vi "Modify Run-Time Menu for Spectral Graph.vi"(7 "spectra info":T1[](array[typedef]) {"x-axis units" items=["Time (s)"=0, "Frequency-CB (Hz)"=1, "Frequency-CPB (Hz)"=1248, "Frequency-Arbitrary (Hz)"=2357, "Quefrency (s)"=2, "Revolutions (rev)"=3, "Order"=4, "Speed (RPM)"=11, "Speed (rad/s)"=21, "Index"=65535]; "weighting filter" items=["Linear", "A-weighting", "B-weighting", "C-weighting", "ITU-R 468-4", "Dolby", "CCITT", "C-message", "Wb", "Wc", "Wd", "We", "Wf", "Wh", "Wj", "Wk", "Wm", "AES17 20 kHz lowpass", "AES17 40 kHz lowpass", "AES17 20 kHz highpass", "AES17 40 kHz highpass"]; "dB reference [EU]" format="%.2f"; "engineering units" items=["custom..."=0, "V"=1, "A"=21, "C"=30, "pC"=31, "s"=32, "-"=29, "Pa"=2, "N"=20, "g"=3, "m/s^2"=4, "m/s"=5, "m"=6, "mm/s"=12, "mm"=13, "micron/s"=14, "micron"=15, "in/s^2"=7, "in/s"=8, "in"=9, "mil/s"=10, "mil"=11, "rad/s^2"=16, "rad/s"=17, "rad"=18, "deg/s^2"=26, "deg/s"=27, "deg"=28, "RPM"=22, "cycle/s^2"=23, "Hz"=24, "cycle"=25, "strain"=19]; "spectral info"."window" items=["None "=0, "Hanning"=1, "Hamming"=2, "Blackman-Harris"=3, "Exact Blackman"=4, "Blackman"=5, "Flat Top"=6, "4 Term B-Harris "=7, "7 Term B-Harris"=8, "Low Sidelobe"=9, "Force - Exponential"=10, "Gaussian"=62]}, 10 "Menu in":refnum<k9>, 11 "Display State In":T7={"Graph Visible Items"={"Plot Legend"=FALSE, "Scale Legend"=FALSE, "Graph Palette"=FALSE, "Cursor Legend"=FALSE, "X Scrollbar"=FALSE}, "View Table"=FALSE, "Table Visible Items"={"Vertical Scrollbar"=FALSE, "Horizontal Scrollbar"=FALSE, "Row Headers"=FALSE, "Column Headers"=FALSE, "Vertical Lines"=FALSE, "Horizontal Lines"=FALSE}, "Header Font"={"Font Name"="", "Size"=0, "Bold"=FALSE, "Italic"=FALSE, "Underline"=FALSE, "Strikeout"=FALSE, "Color"=0}, "Cell Font"={"Font Name"="", "Size"=0, "Bold"=FALSE, "Italic"=FALSE, "Underline"=FALSE, "Strikeout"=FALSE, "Color"=0}, "Description and Tip..."={"Description"="", "Tip"=""}, "Moveable Splitter Position"=0, "Measurement Cursor Configuration"={"XY"={"enable XY"=FALSE, "Position (X)"=[], "Type"=enum."Absolute", "Y reference"=0.0, "color"=0}, "band"={"enable band"=FALSE, "B1"=0.0, "B2"=0.0, "Fixed bandwidth (B2-B1)"=0.0, "B1 color"=0, "B2 color"=0}, "harmonic"={"enable harmonics"=FALSE, "X reference (1X)"=0.0, "Maximum"=0, "Subset"=enum."All", "1X color"=0, "MX color"=0}, "sideband"={"enable sideband"=FALSE, "X center (C)"=0.0, "Sidebands"=0, "X spacing (s)"=0.0, "Center color"=0, "Sideband color"=0}}, "Cursors"={"List"=[], "Tags"=[]}, "X Increment"=0.0, "X Scale"={"Label Visible"=FALSE, "Label Text"="", "Mapping Mode"=0, "Format String"=""}, "Y Scale"={"Label Visible"=FALSE, "Label Text"="", "Mapping Mode"=0, "Format String"=""}, "Colors"={"background"=16777215, "major grid"=8355711, "minor grid"=12632256, "font"=0}, "desired spectrum view"={"scaling"={"linear/dB"=enum."no change", "dB reference"=0.0, "power/magnitude"=enum."no change", "view"=enum."no change"}, "spectral density"=enum."no change"}, "Plot Color Wheel"=[3381759, 32768, 982784, 4375295, 13827953, 13457919, 16757522, 4343295, 16728758, 12095254], "Plots"=[], "registered user events"=variant, "Lock 1X to Peak"=FALSE, "spectrum component"=32, "phase spectrum view"={"desired units"=0, "desired wrapping"=4}} caption="State" {"phase spectrum view"."desired wrapping" items=["No change", "Unwrap", "Wrap: -360 to 0", "Wrap: -270 to 90", "Wrap: -180 to 180", "Wrap: -90 to 270", "Wrap: 0 to 360", "Wrap: custom range"]; "phase spectrum view"."desired units" items=["No change", "Radians", "Degrees", "Cycles"]; "spectrum component" items=["Magnitude^2"=37, "Magnitude"=32, "Phase"=33, "Real"=34, "Imaginary"=35, "Coherence"=36, "Unknown"=99]; "Y Scale"."Mapping Mode" items=["Linear", "Logarithmic", "dB"]; "X Scale"."Mapping Mode" items=["Linear", "Logarithmic"]}) -> (3 "Display State out":T7={"Graph Visible Items"={"Plot Legend"=FALSE, "Scale Legend"=FALSE, "Graph Palette"=FALSE, "Cursor Legend"=FALSE, "X Scrollbar"=FALSE}, "View Table"=FALSE, "Table Visible Items"={"Vertical Scrollbar"=FALSE, "Horizontal Scrollbar"=FALSE, "Row Headers"=FALSE, "Column Headers"=FALSE, "Vertical Lines"=FALSE, "Horizontal Lines"=FALSE}, "Header Font"={"Font Name"="", "Size"=0, "Bold"=FALSE, "Italic"=FALSE, "Underline"=FALSE, "Strikeout"=FALSE, "Color"=0}, "Cell Font"={"Font Name"="", "Size"=0, "Bold"=FALSE, "Italic"=FALSE, "Underline"=FALSE, "Strikeout"=FALSE, "Color"=0}, "Description and Tip..."={"Description"="", "Tip"=""}, "Moveable Splitter Position"=0, "Measurement Cursor Configuration"={"XY"={"enable XY"=FALSE, "Position (X)"=[], "Type"=enum."Absolute", "Y reference"=0.0, "color"=0}, "band"={"enable band"=FALSE, "B1"=0.0, "B2"=0.0, "Fixed bandwidth (B2-B1)"=0.0, "B1 color"=0, "B2 color"=0}, "harmonic"={"enable harmonics"=FALSE, "X reference (1X)"=0.0, "Maximum"=0, "Subset"=enum."All", "1X color"=0, "MX color"=0}, "sideband"={"enable sideband"=FALSE, "X center (C)"=0.0, "Sidebands"=0, "X spacing (s)"=0.0, "Center color"=0, "Sideband color"=0}}, "Cursors"={"List"=[], "Tags"=[]}, "X Increment"=0.0, "X Scale"={"Label Visible"=FALSE, "Label Text"="", "Mapping Mode"=0, "Format String"=""}, "Y Scale"={"Label Visible"=FALSE, "Label Text"="", "Mapping Mode"=0, "Format String"=""}, "Colors"={"background"=16777215, "major grid"=8355711, "minor grid"=12632256, "font"=0}, "desired spectrum view"={"scaling"={"linear/dB"=enum."no change", "dB reference"=0.0, "power/magnitude"=enum."no change", "view"=enum."no change"}, "spectral density"=enum."no change"}, "Plot Color Wheel"=[3381759, 32768, 982784, 4375295, 13827953, 13457919, 16757522, 4343295, 16728758, 12095254], "Plots"=[], "registered user events"=variant, "Lock 1X to Peak"=FALSE, "spectrum component"=32, "phase spectrum view"={"desired units"=0, "desired wrapping"=4}} caption="State" {"phase spectrum view"."desired wrapping" items=["No change", "Unwrap", "Wrap: -360 to 0", "Wrap: -270 to 90", "Wrap: -180 to 180", "Wrap: -90 to 270", "Wrap: 0 to 360", "Wrap: custom range"]; "phase spectrum view"."desired units" items=["No change", "Radians", "Degrees", "Cycles"]; "spectrum component" items=["Magnitude^2"=37, "Magnitude"=32, "Phase"=33, "Real"=34, "Imaginary"=35, "Coherence"=36, "Unknown"=99]; "Y Scale"."Mapping Mode" items=["Linear", "Logarithmic", "dB"]; "X Scale"."Mapping Mode" items=["Linear", "Logarithmic"]})   [LabVIEW 2017, in "Spectrum with Cursors.xctl"]
uses:
  <vilib>/addons/_XControls/Spectrum with Cursors/Spectrum with Cursors.xctl
  <vilib>/addons/_XControls/Spectrum with Cursors/Controls/State.ctl
  <vilib>/Utility/miscctls.llb/LVFontTypeDef.ctl
  <vilib>/addons/_XControls/Spectrum with Cursors/Controls/Measurement Cursor Configuration.ctl
  <vilib>/addons/_NISVFA/_Shared subVIs/Controls/NI Spectrum Component.ctl
  <vilib>/addons/_NISVFA/_Shared subVIs/Controls/svc_Spectrum Info.ctl
  <vilib>/addons/_NISVFA/_Shared subVIs/Controls/svc_X-Axis Units.ctl
  <vilib>/addons/_NISVFA/_Shared subVIs/Controls/svc_Spectrum Type.ctl
  <vilib>/addons/_NISVFA/_Shared subVIs/Controls/svc_Engineering Units Text Ring.ctl
  <vilib>/addons/_NISVFA/_Shared subVIs/Controls/svc_Weighting Filter Text Ring.ctl
  <vilib>/addons/_NISVFA/_Shared subVIs/Controls/svc_Complimentary Spectrum Units.ctl
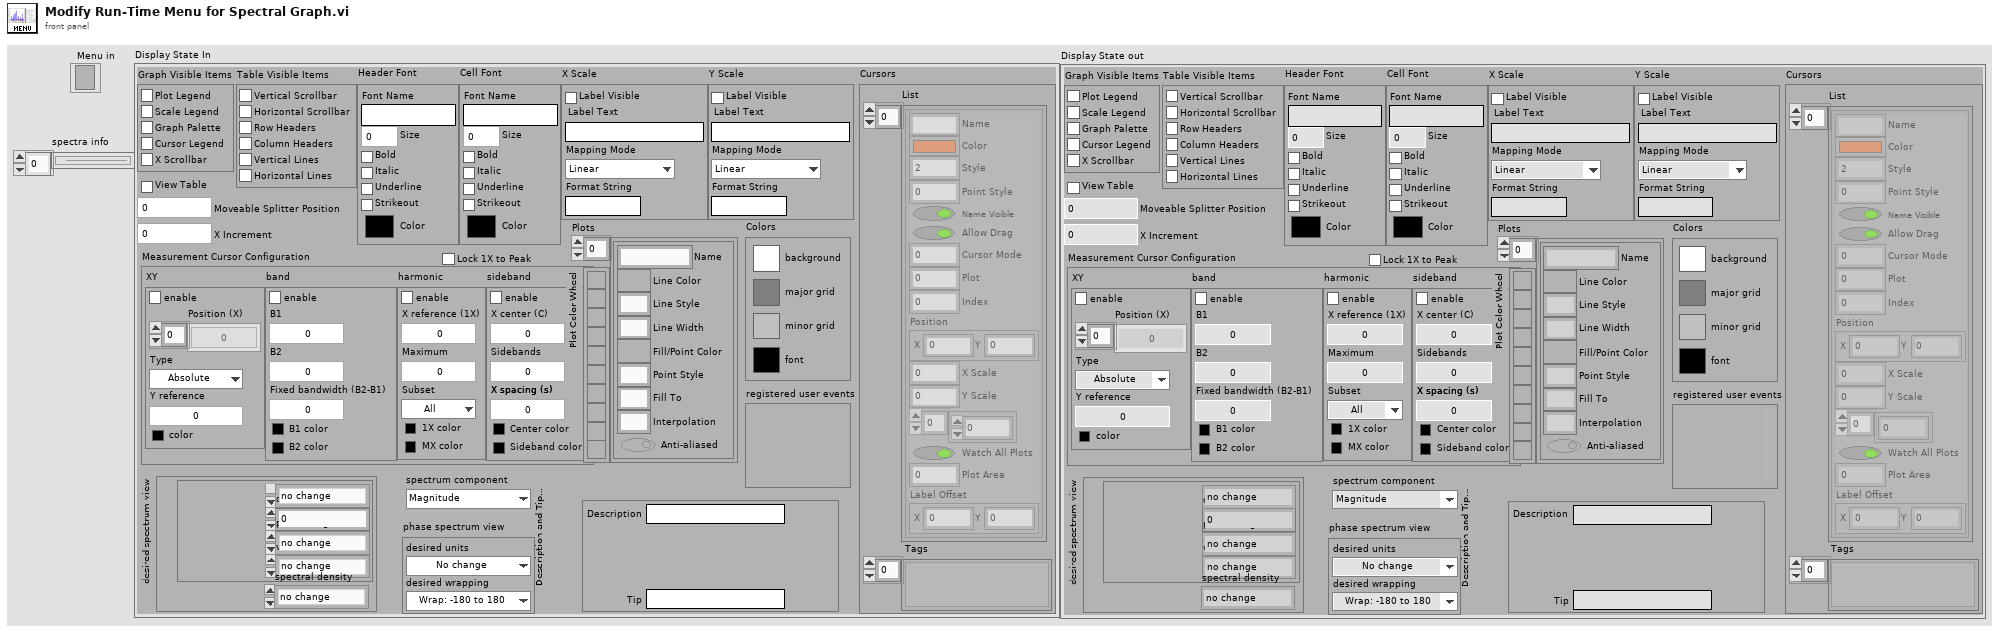
[diagram p1: front panel]
types:
  T1 = typedef "svc_Spectrum Info.ctl" = cluster{"channel name":string, "description":string, "x-axis units":T2, "spectral info":cluster{"spectrum type":T3, "linear/dB":enum16{"linear", "dB"}, "window":u16, "window size":i32, "FFT size":i32}, "engineering units":T4, "custom label":string, "dB reference [EU]":dbl, "peak units":enum16{"rms", "peak", "peak-peak"}, "weighting filter":T5, "spectral density?":bool, "unit label":string, "spectrum skewed?":bool, "complimentary spectrum units":T6}
  T2 = typedef "svc_X-Axis Units.ctl" = u16
  T3 = typedef "svc_Spectrum Type.ctl" = enum16{"FFT Spectrum [complex]", "Amplitude [Magnitude]", "Power [Magnitude^2]", "Cross Spectrum [complex]", "Frequency Response [Complex]"}
  T4 = typedef "svc_Engineering Units Text Ring.ctl" = u16
  T5 = typedef "svc_Weighting Filter Text Ring.ctl" = u16
  T6 = typedef "svc_Complimentary Spectrum Units.ctl" = enum16{"none", "radians", "degrees", "cycles", "imaginary"}
  T7 = typedef "Spectrum with Cursors.xctl/State.ctl" = cluster{"Graph Visible Items":cluster{"Plot Legend":bool, "Scale Legend":bool, "Graph Palette":bool, "Cursor Legend":bool, "X Scrollbar":bool}, "View Table":bool, "Table Visible Items":cluster{"Vertical Scrollbar":bool, "Horizontal Scrollbar":bool, "Row Headers":bool, "Column Headers":bool, "Vertical Lines":bool, "Horizontal Lines":bool}, "Header Font":T8, "Cell Font":T8, "Description and Tip...":cluster{"Description":string, "Tip":string}, "Moveable Splitter Position":i32, "Measurement Cursor Configuration":T9, "Cursors":cluster{"List":cluster{"Name":string, "Color":u32, "Style":i32, "Point Style":u8, "Name Visible":bool, "Allow Drag":bool, "Cursor Mode":u32, "Plot":i32, "Index":i32, "Position":cluster{"X":dbl, "Y":dbl}, "X Scale":u32, "Y Scale":u32, "Watch Plots":i32[], "Watch All Plots":bool, "Plot Area":i32, "Label Offset":cluster{"X":dbl, "Y":dbl}}[], "Tags":variant[]}, "X Increment":dbl, "X Scale":cluster{"Label Visible":bool, "Label Text":string, "Mapping Mode":u8, "Format String":string}, "Y Scale":cluster{"Label Visible":bool, "Label Text":string, "Mapping Mode":u8, "Format String":string}, "Colors":cluster{"background":u32, "major grid":u32, "minor grid":u32, "font":u32}, "desired spectrum view":cluster{"scaling":cluster{"linear/dB":enum16{"no change", "linear", "dB"}, "dB reference":dbl, "power/magnitude":enum16{"no change", "power", "magnitude"}, "view":enum16{"no change", "rms", "peak", "peak-peak"}}, "spectral density":enum16{"no change", "spectrum", "spectral density"}}, "Plot Color Wheel":u32[], "Plots":cluster{"Name":string, "Line Color":u32, "Line Style":u8, "Line Width":u8, "Fill/Point Color":u32, "Point Style":u8, "Fill To":i16, "Interpolation":u8, "Anti-aliased":bool}[], "registered user events":variant, "Lock 1X to Peak":bool, "spectrum component":T10, "phase spectrum view":cluster{"desired units":u16, "desired wrapping":u16}}
  T8 = typedef "LVFontTypeDef.ctl" = cluster{"Font Name":string, "Size":u16, "Bold":bool, "Italic":bool, "Underline":bool, "Strikeout":bool, "Color":u32}
  T9 = typedef "Spectrum with Cursors.xctl/Measurement Cursor Configuration.ctl" = cluster{"XY":cluster{"enable XY":bool, "Position (X)":dbl[], "Type":enum16{"Absolute", "Relative"}, "Y reference":dbl, "color":u32}, "band":cluster{"enable band":bool, "B1":dbl, "B2":dbl, "Fixed bandwidth (B2-B1)":dbl, "B1 color":u32, "B2 color":u32}, "harmonic":cluster{"enable harmonics":bool, "X reference (1X)":dbl, "Maximum":i32, "Subset":enum16{"All", "Even", "Odd"}, "1X color":u32, "MX color":u32}, "sideband":cluster{"enable sideband":bool, "X center (C)":dbl, "Sidebands":i32, "X spacing (s)":dbl, "Center color":u32, "Sideband color":u32}}
  T10 = typedef "NI Spectrum Component.ctl" = u16
  T11 = enum16{"no change", "spectrum", "spectral density"}
  T12 = enum16{"No change", "Radians", "Degrees", "Cycles"}
  T13 = enum16{"No change", "Unwrap", "Wrap: -360 to 0", "Wrap: -270 to 90", "Wrap: -180 to 180", "Wrap: -90 to 270", "Wrap: 0 to 360", "Wrap: custom range"}
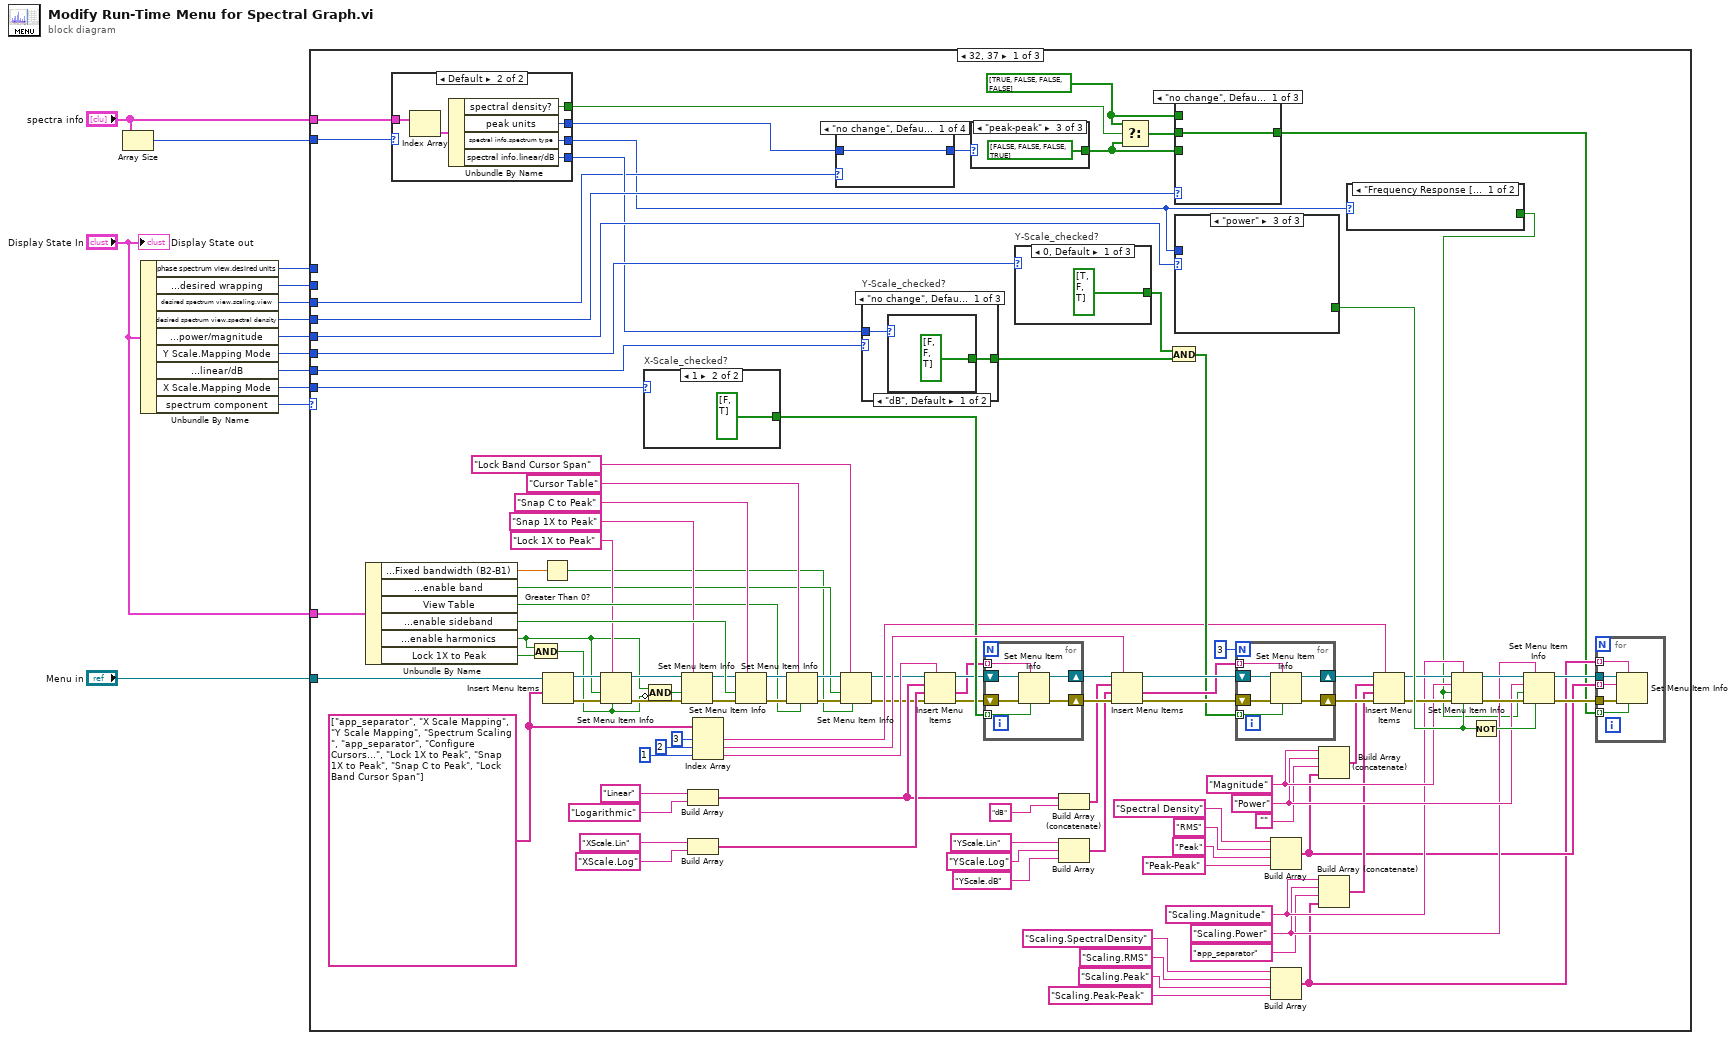
[diagram p0: block diagram]
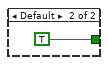
[diagram p2: hidden frame]
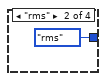
[diagram p3: hidden frame]
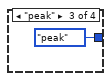
[diagram p4: hidden frame]
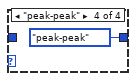
[diagram p5: hidden frame]
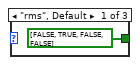
[diagram p6: hidden frame]
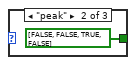
[diagram p7: hidden frame]
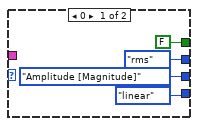
[diagram p8: hidden frame]
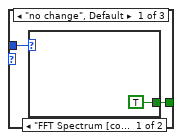
[diagram p11: hidden frame]
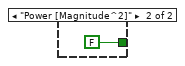
[diagram p12: hidden frame]
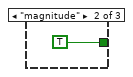
[diagram p13: hidden frame]
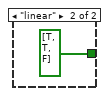
[diagram p14: hidden frame]
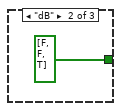
[diagram p15: hidden frame]
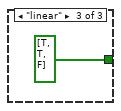
[diagram p16: hidden frame]
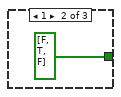
[diagram p17: hidden frame]
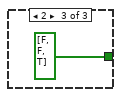
[diagram p18: hidden frame]
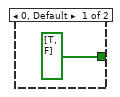
[diagram p19: hidden frame]
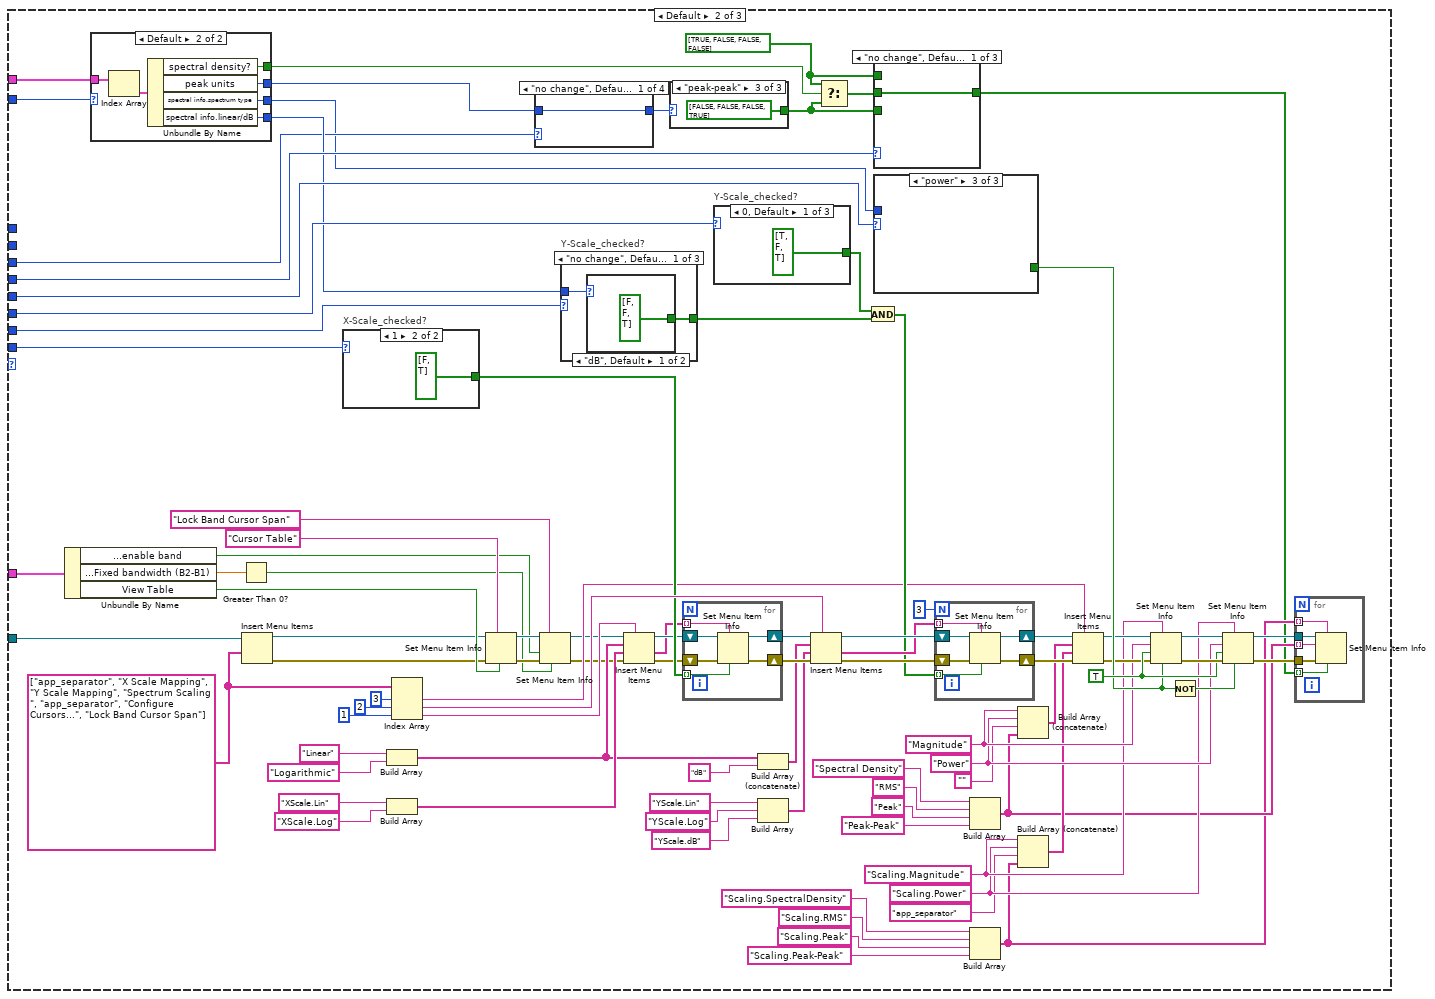
[diagram p20: hidden frame]
diagram:
  n1 = Array Size(array="spectra info") -> (size(s)=w6:i32)
  n2 = Unbundle By Name("Display State In") -> ("phase spectrum view.desired units"=w2:u16, "phase spectrum view.desired wrapping"=w1:u16, "desired spectrum view.scaling.view"=w4:enum16{"no change", "rms", "peak", "peak-peak"}, "desired spectrum view.spectral density"=w7:T11, "desired spectrum view.scaling.power/magnitude"=w8:enum16{"no change", "power", "magnitude"}, "Y Scale.Mapping Mode"=w10:u8, "desired spectrum view.scaling.linear/dB"=w9:enum16{"no change", "linear", "dB"}, "X Scale.Mapping Mode"=w12:u8, "spectrum component"=w3:T10)
  n3 = case shown="32, 37" w3 {
    tunnel: "Menu in" -> [w112 w265 w386]
    tunnel: w12 -> [w103 w256 w377]
    tunnel: "Display State In" -> [w97 w250 w371]
    tunnel: w10 -> [w96 w249 _]
    tunnel: w9 -> [w80 w233 _]
    tunnel: w8 -> [w64 w225 _]
    tunnel: w7 -> [w45 w206 _]
    tunnel: w6 -> [w44 w205 w336]
    tunnel: "spectra info" -> [w43 w204 w337]
    tunnel: w4 -> [w27 w188 _]
    tunnel: w2 -> [_ _ w322]
    tunnel: w1 -> [_ _ w324]
    frame 32, 37 {
      w29 = bool[] [TRUE, FALSE, FALSE, FALSE]
      w51 = "Scaling.Power"
      w52 = "Scaling.Magnitude"
      w54 = "Power" ("element")
      w55 = "Magnitude" ("element")
      w107 = string[] ["app_separator", "X Scale Mapping", "Y Scale Mapping", "Spectrum Scaling ", "app_separator", "Configure Cursors...", "Lock 1X to Peak", "Snap 1X to Peak", "Snap C to Peak", "Lock Band Cursor Span"]
      n4 = Unbundle By Name(w97) -> ("Measurement Cursor Configuration.band.Fixed bandwidth (B2-B1)"=w17:dbl, "Measurement Cursor Configuration.band.enable band"=w18:bool, "View Table"=w110:bool, "Measurement Cursor Configuration.sideband.enable sideband"=w119:bool, "Measurement Cursor Configuration.harmonic.enable harmonics"=w69:bool, "Lock 1X to Peak"=w71:bool)
      n5 = case shown="Default" w44 {
        tunnel: w43 -> [_ w142]
        tunnel: [enum16{"rms", "peak", "peak-peak"}."rms" ("peak units") w140] -> w26
        tunnel: [FALSE ("spectral density?") w137] -> w30
        tunnel: [svc_Spectrum_Type."Amplitude [Magnitude]" ("spectrum type") w139] -> w15
        tunnel: [enum16{"linear", "dB"}."linear" ("linear/dB") w138] -> w42
        frame 0 {
        }
        frame Default {
          n6 = Index Array(array=w142) -> (element=w141:T1)  [unwired: 1 in]
          n7 = Unbundle By Name(w141) -> ("spectral density?"=w137:bool, "peak units"=w140:enum16{"rms", "peak", "peak-peak"}, "spectral info.spectrum type"=w139:T3, "spectral info.linear/dB"=w138:enum16{"linear", "dB"})
        }
      }
      n8 = And(x=w69, y=w71) -> (x .and. y?=w70:bool)
      n9 = Greater Than 0?(x=w17) -> (x > 0?=w16:bool)
      n10 = Insert Menu Items(7:w107, 9:w112) -> (0:w73:errorcluster, 3:w74:refnum<k9>)  [unwired: 4 in, 1 out]
      n11 = Set Menu Item Info(6:w70, 7:"Lock 1X to Peak", 8:w73, 9:w69, 11:w74) -> (0:w76:errorcluster, 3:w75:refnum<k9>)  [unwired: 2 in]
      n12 = case "X-Scale_checked?" shown="1" w103 {
        tunnel: [bool[] [TRUE, FALSE] bool[] [FALSE, TRUE]] -> w95
        frame 0, Default {
        }
        frame 1 {
        }
      }
      n13 = Compound Arithmetic op=AND(w69, invert w70) -> (w68:bool)
      n14 = Set Menu Item Info(7:"Snap 1X to Peak", 8:w76, 9:w68, 11:w75) -> (0:w116:errorcluster, 3:w113:refnum<k9>)  [unwired: 3 in]
      n15 = Build Array("Linear", "Logarithmic") -> (w84:string[])
      n16 = Build Array("XScale.Lin", "XScale.Log") -> (w89:string[])
      n17 = Index Array(array=w107, index #1=3 ("index"), index #2=2 ("index"), index #3=1 ("index")) -> (element #1=w56:string, element #2=w104:string, element #3=w92:string)
      n18 = Set Menu Item Info(7:"Snap C to Peak", 8:w116, 9:w119, 11:w113) -> (0:w115:errorcluster, 3:w114:refnum<k9>)  [unwired: 3 in]
      n19 = Set Menu Item Info(6:w110, 7:"Cursor Table", 8:w115, 11:w114) -> (0:w23:errorcluster, 3:w22:refnum<k9>)  [unwired: 3 in]
      n20 = case shown="\"no change\", Default" w27 {
        tunnel: w26 -> [w121 _ _ _]
        tunnel: [w121 enum16{"rms", "peak", "peak-peak"}."rms" ("peak units") enum16{"rms", "peak", "peak-peak"}."peak" ("peak units") enum16{"rms", "peak", "peak-peak"}."peak-peak" ("peak units")] -> w25
        frame "no change", Default {
        }
        frame "rms" {
        }
        frame "peak" {
        }
        frame "peak-peak" {
        }
      }
      n21 = Set Menu Item Info(6:w16, 7:"Lock Band Cursor Span", 8:w23, 9:w18, 11:w22) -> (0:w20:errorcluster, 3:w21:refnum<k9>)  [unwired: 2 in]
      n22 = case "Y-Scale_checked?" shown="\"no change\", Default" w80 {
        tunnel: [w152 bool[] [FALSE, FALSE, TRUE] bool[] [TRUE, TRUE, FALSE]] -> w79
        tunnel: w42 -> [w151 _ _]
        frame "no change", Default {
          n23 = case shown="\"dB\", Default" w151 {
            tunnel: [bool[] [FALSE, FALSE, TRUE] bool[] [TRUE, TRUE, FALSE]] -> w152
            frame "dB", Default {
            }
            frame "linear" {
            }
          }
        }
        frame "dB" {
        }
        frame "linear" {
        }
      }
      n24 = Insert Menu Items(5:w92, 6:w20, 7:w89, 8:w84, 9:w21) -> (0:w93:errorcluster, 1:w88:string[], 3:w94:refnum<k9>)  [unwired: 1 in]
      n25 = case shown="\"peak-peak\"" w25 {
        tunnel: [bool[] [FALSE, TRUE, FALSE, FALSE] bool[] [FALSE, FALSE, TRUE, FALSE] bool[] [FALSE, FALSE, FALSE, TRUE]] -> w24
        frame "rms", Default {
        }
        frame "peak" {
        }
        frame "peak-peak" {
        }
      }
      n26 = for {
        shift-right: [w166] -> w101
        shift-left: w94 -> [w168]
        shift-right: [w165] -> w102
        shift-left: w93 -> [w167]
        tunnel: w95 -> [w164] mode=indexing
        tunnel: w88 -> [w163] mode=indexing
        n27 = Set Menu Item Info(6:w164, 7:w163, 8:w167, 11:w168) -> (0:w165:errorcluster, 3:w166:refnum<k9>)  [unwired: 3 in]
      }
      n28 = case "Y-Scale_checked?" shown="0, Default" w96 {
        tunnel: [bool[] [TRUE, FALSE, TRUE] bool[] [FALSE, TRUE, FALSE] bool[] [FALSE, FALSE, TRUE]] -> w77
        frame 0, Default {
        }
        frame 1 {
        }
        frame 2 {
        }
      }
      n29 = Build Array (concatenate)(w84, "dB") -> (w83:string[])
      n30 = Build Array("YScale.Lin", "YScale.Log", "YScale.dB") -> (w85:string[])
      n31 = Insert Menu Items(5:w104, 6:w102, 7:w85, 8:w83, 9:w101) -> (0:w99:errorcluster, 1:w98:string[], 3:w100:refnum<k9>)  [unwired: 1 in]
      n32 = Select(t=w29, s=w30, f=w24) -> (s? t:f=w28:bool[])
      n33 = And(x=w77, y=w79) -> (x .and. y?=w78:bool[])
      n34 = case shown="\"no change\", Default" w45 {
        tunnel: [w143 w144 w145] -> w31
        tunnel: w29 -> [_ _ w145]
        tunnel: w28 -> [w143 _ _]
        tunnel: w24 -> [_ w144 _]
        frame "no change", Default {
        }
        frame "spectrum" {
        }
        frame "spectral density" {
        }
      }
      n35 = case shown="\"power\"" w64 {
        tunnel: [w147 TRUE ("enabled") _] -> w63
        tunnel: w15 -> [w146 _ _]
        frame "no change", Default {
          n36 = case shown="\"FFT Spectrum [complex]\", \"Amplitude [Magnitude]\", Default" w146 {
            tunnel: [TRUE ("enabled") FALSE ("enabled")] -> w147
            frame "FFT Spectrum [complex]", "Amplitude [Magnitude]", Default {
            }
            frame "Power [Magnitude^2]" {
            }
          }
        }
        frame "magnitude" {
        }
        frame "power" {
        }
      }
      n37 = for {
        N: 3 -> [_]
        shift-right: [w160] -> w59
        shift-left: w100 -> [w162]
        tunnel: w98 -> [w159] mode=indexing
        shift-right: [w158] -> w60
        shift-left: w99 -> [w161]
        tunnel: w78 -> [w157] mode=indexing
        n38 = Set Menu Item Info(6:w157, 7:w159, 8:w161, 11:w162) -> (0:w158:errorcluster, 3:w160:refnum<k9>)  [unwired: 3 in]
      }
      n39 = Build Array("Spectral Density" ("element"), "RMS" ("element"), "Peak" ("element"), "Peak-Peak" ("element")) -> (w33:string[])
      n40 = Build Array("Scaling.SpectralDensity", "Scaling.RMS", "Scaling.Peak", "Scaling.Peak-Peak") -> (w32:string[])
      n41 = Build Array (concatenate)(w55, w54, "" ("element"), w33) -> (w53:string[])
      n42 = Build Array (concatenate)(w52, w51, "app_separator", w32) -> (w50:string[])
      n43 = case shown="\"Frequency Response [Complex]\"" w15 {
        tunnel: [_ TRUE ("enabled")] -> w14
        frame "Frequency Response [Complex]" {
        }
        frame Default {
        }
      }
      n44 = Insert Menu Items(5:w56, 6:w60, 7:w50, 8:w53, 9:w59) -> (0:w58:errorcluster, 3:w57:refnum<k9>)  [unwired: 1 in, 1 out]
      n45 = Set Menu Item Info(6:w63, 7:w52, 8:w58, 9:w14, 10:w55, 11:w57) -> (0:w65:errorcluster, 3:w66:refnum<k9>)  [unwired: 1 in]
      n46 = Not(x=w63) -> (.not. x?=w62:bool)
      n47 = Set Menu Item Info(6:w62, 7:w51, 8:w65, 9:w14, 10:w54, 11:w66) -> (0:w47:errorcluster, 3:w46:refnum<k9>)  [unwired: 1 in]
      n48 = for {
        tunnel: w47 -> [w132]
        tunnel: w46 -> [w131]
        tunnel: w33 -> [w130] mode=indexing
        tunnel: w32 -> [w129] mode=indexing
        tunnel: w31 -> [w128] mode=indexing
        n49 = Set Menu Item Info(6:w128, 7:w129, 8:w132, 10:w130, 11:w131) -> ()  [unwired: 2 in, 2 out]
      }
    }
    frame Default {
      w190 = bool[] [TRUE, FALSE, FALSE, FALSE]
      w226 = TRUE ("enabled")
      w212 = "Scaling.Power"
      w213 = "Scaling.Magnitude"
      w215 = "Power" ("element")
      w216 = "Magnitude" ("element")
      w260 = string[] ["app_separator", "X Scale Mapping", "Y Scale Mapping", "Spectrum Scaling ", "app_separator", "Configure Cursors...", "Lock Band Cursor Span"]
      n50 = Unbundle By Name(w250) -> ("Measurement Cursor Configuration.band.enable band"=w174:bool, "Measurement Cursor Configuration.band.Fixed bandwidth (B2-B1)"=w178:dbl, "View Table"=w263:bool)
      n51 = case shown="Default" w205 {
        tunnel: w204 -> [_ w287]
        tunnel: [enum16{"rms", "peak", "peak-peak"}."rms" ("peak units") w285] -> w186
        tunnel: [FALSE ("spectral density?") w282] -> w191
        tunnel: [svc_Spectrum_Type."Amplitude [Magnitude]" ("spectrum type") w284] -> w187
        tunnel: [enum16{"linear", "dB"}."linear" ("linear/dB") w283] -> w203
        frame 0 {
        }
        frame Default {
          n52 = Index Array(array=w287) -> (element=w286:T1)  [unwired: 1 in]
          n53 = Unbundle By Name(w286) -> ("spectral density?"=w282:bool, "peak units"=w285:enum16{"rms", "peak", "peak-peak"}, "spectral info.spectrum type"=w284:T3, "spectral info.linear/dB"=w283:enum16{"linear", "dB"})
        }
      }
      n54 = Greater Than 0?(x=w178) -> (x > 0?=w177:bool)
      n55 = Insert Menu Items(7:w260, 9:w265) -> (0:w175:errorcluster, 3:w176:refnum<k9>)  [unwired: 4 in, 1 out]
      n56 = case "X-Scale_checked?" shown="1" w256 {
        tunnel: [bool[] [TRUE, FALSE] bool[] [FALSE, TRUE]] -> w248
        frame 0, Default {
        }
        frame 1 {
        }
      }
      n57 = Build Array("Linear", "Logarithmic") -> (w237:string[])
      n58 = Build Array("XScale.Lin", "XScale.Log") -> (w242:string[])
      n59 = Index Array(array=w260, index #1=3 ("index"), index #2=2 ("index"), index #3=1 ("index")) -> (element #1=w217:string, element #2=w257:string, element #3=w245:string)
      n60 = Set Menu Item Info(6:w263, 7:"Cursor Table", 8:w175, 11:w176) -> (0:w183:errorcluster, 3:w182:refnum<k9>)  [unwired: 3 in]
      n61 = case shown="\"no change\", Default" w188 {
        tunnel: w186 -> [w266 _ _ _]
        tunnel: [w266 enum16{"rms", "peak", "peak-peak"}."rms" ("peak units") enum16{"rms", "peak", "peak-peak"}."peak" ("peak units") enum16{"rms", "peak", "peak-peak"}."peak-peak" ("peak units")] -> w185
        frame "no change", Default {
        }
        frame "rms" {
        }
        frame "peak" {
        }
        frame "peak-peak" {
        }
      }
      n62 = Set Menu Item Info(6:w177, 7:"Lock Band Cursor Span", 8:w183, 9:w174, 11:w182) -> (0:w180:errorcluster, 3:w181:refnum<k9>)  [unwired: 2 in]
      n63 = case "Y-Scale_checked?" shown="\"no change\", Default" w233 {
        tunnel: [w297 bool[] [FALSE, FALSE, TRUE] bool[] [TRUE, TRUE, FALSE]] -> w232
        tunnel: w203 -> [w296 _ _]
        frame "no change", Default {
          n64 = case shown="\"dB\", Default" w296 {
            tunnel: [bool[] [FALSE, FALSE, TRUE] bool[] [TRUE, TRUE, FALSE]] -> w297
            frame "dB", Default {
            }
            frame "linear" {
            }
          }
        }
        frame "dB" {
        }
        frame "linear" {
        }
      }
      n65 = Insert Menu Items(5:w245, 6:w180, 7:w242, 8:w237, 9:w181) -> (0:w246:errorcluster, 1:w241:string[], 3:w247:refnum<k9>)  [unwired: 1 in]
      n66 = case shown="\"peak-peak\"" w185 {
        tunnel: [bool[] [FALSE, TRUE, FALSE, FALSE] bool[] [FALSE, FALSE, TRUE, FALSE] bool[] [FALSE, FALSE, FALSE, TRUE]] -> w184
        frame "rms", Default {
        }
        frame "peak" {
        }
        frame "peak-peak" {
        }
      }
      n67 = for {
        shift-right: [w311] -> w254
        shift-left: w247 -> [w313]
        shift-right: [w310] -> w255
        shift-left: w246 -> [w312]
        tunnel: w248 -> [w309] mode=indexing
        tunnel: w241 -> [w308] mode=indexing
        n68 = Set Menu Item Info(6:w309, 7:w308, 8:w312, 11:w313) -> (0:w310:errorcluster, 3:w311:refnum<k9>)  [unwired: 3 in]
      }
      n69 = case "Y-Scale_checked?" shown="0, Default" w249 {
        tunnel: [bool[] [TRUE, FALSE, TRUE] bool[] [FALSE, TRUE, FALSE] bool[] [FALSE, FALSE, TRUE]] -> w230
        frame 0, Default {
        }
        frame 1 {
        }
        frame 2 {
        }
      }
      n70 = Build Array (concatenate)(w237, "dB") -> (w236:string[])
      n71 = Build Array("YScale.Lin", "YScale.Log", "YScale.dB") -> (w238:string[])
      n72 = Insert Menu Items(5:w257, 6:w255, 7:w238, 8:w236, 9:w254) -> (0:w252:errorcluster, 1:w251:string[], 3:w253:refnum<k9>)  [unwired: 1 in]
      n73 = Select(t=w190, s=w191, f=w184) -> (s? t:f=w189:bool[])
      n74 = And(x=w230, y=w232) -> (x .and. y?=w231:bool[])
      n75 = case shown="\"no change\", Default" w206 {
        tunnel: [w288 w289 w290] -> w192
        tunnel: w190 -> [_ _ w290]
        tunnel: w189 -> [w288 _ _]
        tunnel: w184 -> [_ w289 _]
        frame "no change", Default {
        }
        frame "spectrum" {
        }
        frame "spectral density" {
        }
      }
      n76 = case shown="\"power\"" w225 {
        tunnel: [w292 TRUE ("enabled") _] -> w224
        tunnel: w187 -> [w291 _ _]
        frame "no change", Default {
          n77 = case shown="\"FFT Spectrum [complex]\", \"Amplitude [Magnitude]\", Default" w291 {
            tunnel: [TRUE ("enabled") FALSE ("enabled")] -> w292
            frame "FFT Spectrum [complex]", "Amplitude [Magnitude]", Default {
            }
            frame "Power [Magnitude^2]" {
            }
          }
        }
        frame "magnitude" {
        }
        frame "power" {
        }
      }
      n78 = for {
        N: 3 -> [_]
        shift-right: [w305] -> w220
        shift-left: w253 -> [w307]
        tunnel: w251 -> [w304] mode=indexing
        shift-right: [w303] -> w221
        shift-left: w252 -> [w306]
        tunnel: w231 -> [w302] mode=indexing
        n79 = Set Menu Item Info(6:w302, 7:w304, 8:w306, 11:w307) -> (0:w303:errorcluster, 3:w305:refnum<k9>)  [unwired: 3 in]
      }
      n80 = Build Array("Spectral Density" ("element"), "RMS" ("element"), "Peak" ("element"), "Peak-Peak" ("element")) -> (w194:string[])
      n81 = Build Array("Scaling.SpectralDensity", "Scaling.RMS", "Scaling.Peak", "Scaling.Peak-Peak") -> (w193:string[])
      n82 = Build Array (concatenate)(w216, w215, "" ("element"), w194) -> (w214:string[])
      n83 = Build Array (concatenate)(w213, w212, "app_separator", w193) -> (w211:string[])
      n84 = Insert Menu Items(5:w217, 6:w221, 7:w211, 8:w214, 9:w220) -> (0:w219:errorcluster, 3:w218:refnum<k9>)  [unwired: 1 in, 1 out]
      n85 = Set Menu Item Info(6:w224, 7:w213, 8:w219, 9:w226, 10:w216, 11:w218) -> (0:w227:errorcluster, 3:w228:refnum<k9>)  [unwired: 1 in]
      n86 = Not(x=w224) -> (.not. x?=w223:bool)
      n87 = Set Menu Item Info(6:w223, 7:w212, 8:w227, 9:w226, 10:w215, 11:w228) -> (0:w208:errorcluster, 3:w207:refnum<k9>)  [unwired: 1 in]
      n88 = for {
        tunnel: w208 -> [w277]
        tunnel: w207 -> [w276]
        tunnel: w194 -> [w275] mode=indexing
        tunnel: w193 -> [w274] mode=indexing
        tunnel: w192 -> [w273] mode=indexing
        n89 = Set Menu Item Info(6:w273, 7:w274, 8:w277, 10:w275, 11:w276) -> ()  [unwired: 2 in, 2 out]
      }
    }
    frame 33 {
      (unwired) T12."Cycles" ("desired units")
      (unwired) T13."No change" ("desired wrapping")
      w381 = string[] ["app_separator", "X Scale Mapping", "Phase Wrapping", "Phase Units", "app_separator", "Configure Cursors...", "Lock Band Cursor Span"]
      n90 = case shown="Default" w336 {
        tunnel: w337 -> [_ w405]
        tunnel: [_ w403] -> w321
        tunnel: [_ w401] -> w320
        frame 0 {
        }
        frame Default {
          (unwired) svc_Complimentary_Spectrum_Units."none" ("complimentary spectrum units")
          n91 = Index Array(array=w405) -> (element=w404:T1)  [unwired: 1 in]
          n92 = Unbundle By Name(w404) -> ("complimentary spectrum units"=w402:T6)
          n93 = case shown="\"none\"" w402 {
            tunnel: w404 -> [_ w412 w417]
            tunnel: [_ w410 _] -> w403
            frame "none" {
            }
            frame "radians".."cycles" {
              n94 = call <vilib>:"sfva_Get SV Info from Spectrum Info Description.vi"("spectrum info"=w412) -> ("SV Info"=w414:variant, "error out"=w413:errorcluster)  [unwired: 10 in, 3 out]
              n95 = Get Variant Attribute(Variant=w414, name="NI_PhaseUnwrapped", default value (empty Variant)=FALSE ("replaced"), error in=w413) -> (value=w410:bool)  [unwired: 3 out]
            }
            frame Default {
              n96 = call <vilib>:"sfva_Get SV Info from Spectrum Info Description.vi"("spectrum info"=w417) -> ("spectrum info"=w424:T1, "description"=w423:string, "SV Info"=w419:variant, "error out"=w418:errorcluster)  [unwired: 10 in, 1 out]
              n97 = Set Variant Attribute(Variant=w419, name="NI_PhaseUnwrapped", value=FALSE ("replaced"), error in=w418) -> (Variant out=w420:variant, error out=w421:errorcluster)  [unwired: 1 out]
              n98 = call <vilib>:"sfva_Set SV Info in Spectrum Info Description.vi"("spectrum info"=w424, "description"=w423, "SV Info"=w420, "error in (no error)"=w421) -> ()  [unwired: 10 in, 2 out]
            }
          }
          n99 = case shown="\"degrees\"" w402 {
            tunnel: [bool[] [FALSE, TRUE, FALSE] bool[] [TRUE, FALSE, FALSE] bool[] [FALSE, FALSE, TRUE] bool[] [FALSE, FALSE, FALSE]] -> w401
            frame "radians" {
            }
            frame "degrees" {
            }
            frame "cycles" {
            }
            frame Default {
            }
          }
        }
      }
      n100 = Unbundle By Name(w371) -> ("Measurement Cursor Configuration.band.enable band"=w335:bool, "Measurement Cursor Configuration.band.Fixed bandwidth (B2-B1)"=w339:dbl, "View Table"=w384:bool)
      n101 = Greater Than 0?(x=w339) -> (x > 0?=w338:bool)
      n102 = Insert Menu Items(7:w381, 9:w386) -> (0:w355:errorcluster, 3:w356:refnum<k9>)  [unwired: 4 in, 1 out]
      n103 = Set Menu Item Info(6:w384, 7:"Cursor Table", 8:w355, 11:w356) -> (0:w344:errorcluster, 3:w343:refnum<k9>)  [unwired: 3 in]
      n104 = case "X-Scale_checked?" shown="1" w377 {
        tunnel: [bool[] [TRUE, FALSE] bool[] [FALSE, TRUE]] -> w370
        frame 0, Default {
        }
        frame 1 {
        }
      }
      n105 = Set Menu Item Info(6:w338, 7:"Lock Band Cursor Span", 8:w344, 9:w335, 11:w343) -> (0:w341:errorcluster, 3:w342:refnum<k9>)  [unwired: 2 in]
      n106 = Build Array("Linear", "Logarithmic") -> (w359:string[])
      n107 = Build Array("XScale.Lin", "XScale.Log") -> (w364:string[])
      n108 = Index Array(array=w381, index #1=3 ("index"), index #2=2 ("index"), index #3=1 ("index")) -> (element #1=w328:string, element #2=w378:string, element #3=w367:string)
      n109 = case shown="6" w324 {
        tunnel: [bool[] [FALSE, FALSE, FALSE, FALSE] w393 bool[] [FALSE, FALSE, FALSE, TRUE] bool[] [TRUE, FALSE, FALSE, FALSE] bool[] [FALSE, TRUE, FALSE, FALSE] bool[] [FALSE, FALSE, TRUE, FALSE]] -> w323
        tunnel: w321 -> [_ w395 _ _ _ _]
        frame Default {
        }
        frame 0 {
          n110 = Select(t=bool[] [FALSE, FALSE, FALSE, TRUE], s=w395, f=bool[] [FALSE, FALSE, FALSE, FALSE]) -> (s? t:f=w393:bool[])
        }
        frame 1 {
        }
        frame 2 {
        }
        frame 4 {
        }
        frame 6 {
        }
      }
      n111 = Insert Menu Items(5:w367, 6:w341, 7:w364, 8:w359, 9:w342) -> (0:w368:errorcluster, 1:w363:string[], 3:w369:refnum<k9>)  [unwired: 1 in]
      n112 = for {
        shift-right: [w439] -> w375
        shift-left: w369 -> [w441]
        shift-right: [w438] -> w376
        shift-left: w368 -> [w440]
        tunnel: w370 -> [w437] mode=indexing
        tunnel: w363 -> [w436] mode=indexing
        n113 = Set Menu Item Info(6:w437, 7:w436, 8:w440, 11:w441) -> (0:w438:errorcluster, 3:w439:refnum<k9>)  [unwired: 3 in]
      }
      n114 = Build Array("Wrap Phase: -360 to 0", "Wrap Phase: -180 to 180", "Wrap Phase: 0 to 360", "Unwrap Phase") -> (w358:string[])
      n115 = Build Array("Phase.-360to0", "Phase.-180to180", "Phase.0to360", "Phase.Unwrap") -> (w360:string[])
      n116 = case shown="3" w322 {
        tunnel: [bool[] [FALSE, FALSE, FALSE, FALSE] w388 bool[] [TRUE, FALSE, FALSE] bool[] [FALSE, TRUE, FALSE] bool[] [FALSE, FALSE, TRUE]] -> w319
        tunnel: w320 -> [_ w388 _ _ _]
        frame Default {
        }
        frame 0 {
        }
        frame 2 {
        }
        frame 1 {
        }
        frame 3 {
        }
      }
      n117 = Insert Menu Items(5:w378, 6:w376, 7:w360, 8:w358, 9:w375) -> (0:w373:errorcluster, 1:w372:string[], 3:w374:refnum<k9>)  [unwired: 1 in]
      n118 = for {
        N: 4 -> [_]
        shift-right: [w433] -> w352
        shift-left: w374 -> [w435]
        tunnel: w372 -> [w432] mode=indexing
        shift-right: [w431] -> w353
        shift-left: w373 -> [w434]
        tunnel: w323 -> [w430] mode=indexing
        n119 = Set Menu Item Info(6:w430, 7:w432, 8:w434, 11:w435) -> (0:w431:errorcluster, 3:w433:refnum<k9>)  [unwired: 3 in]
      }
      n120 = Build Array("Scaling.Degrees", "Scaling.Radians", "Scaling.Cycles") -> (w326:string[])
      n121 = Build Array("Degrees" ("element"), "Radians" ("element"), "Cycles" ("element")) -> (w325:string[])
      n122 = Insert Menu Items(5:w328, 6:w353, 7:w326, 8:w325, 9:w352) -> (0:w351:errorcluster, 3:w350:refnum<k9>)  [unwired: 1 in, 1 out]
      n123 = for {
        tunnel: w351 -> [w429]
        tunnel: w350 -> [w428]
        tunnel: w325 -> [w427] mode=indexing
        tunnel: w326 -> [w426] mode=indexing
        tunnel: w319 -> [w425] mode=indexing
        n124 = Set Menu Item Info(6:w425, 7:w426, 8:w429, 10:w427, 11:w428) -> ()  [unwired: 2 in, 2 out]
      }
    }
  }
  "Display State out" <- "Display State In"
